vi "SPARK Set Parameter Byte Array.vi"(8 "error in (no error)":errorcluster, 9 "Bytes LSB First":u8[](array[numeric]), 10 "Parameter ID":T6, 11 "MotorControlDeviceRef":T1={"DeviceStatus"={"status"=FALSE, "code"=0, "source"=""}, "Type"=enum."CAN", "PWM"={"PWM Channel"=enum."Invalid", "DeadBand"={"Name"="", "maxPositivePwm"=0, "minPositivePwm"=0, "centerPwm"=0, "maxNegativePwm"=0, "minNegativePwm"=0, "angularRange"=0}}, "CAN"={"Device Number"=8, "SetOutput VI Ref"=variant, "GetOutput VI Ref"=variant, "Enable VI Ref"=variant, "Disable VI Ref"=variant, "Data"=variant(cluster{"Ext ID":u32, "Motor Type":enum16{"Brushed", "Brushless"}} {"Ext ID"=33882120, "Motor Type"=enum."Brushed"})}, "Invert"=FALSE, "DIO PWM"={"PWM \"Enable\" Channel"=enum."Invalid", "DIOChannel"=enum."Invalid", "PWM Rate"=0.0}}) -> (0 "error out":errorcluster, 3 "MotorControlDeviceRef":T1={"DeviceStatus"={"status"=FALSE, "code"=0, "source"=""}, "Type"=enum."CAN", "PWM"={"PWM Channel"=enum."Invalid", "DeadBand"={"Name"="", "maxPositivePwm"=0, "minPositivePwm"=0, "centerPwm"=0, "maxNegativePwm"=0, "minNegativePwm"=0, "angularRange"=0}}, "CAN"={"Device Number"=8, "SetOutput VI Ref"=variant, "GetOutput VI Ref"=variant, "Enable VI Ref"=variant, "Disable VI Ref"=variant, "Data"=variant(cluster{"Ext ID":u32, "Motor Type":enum16{"Brushed", "Brushless"}} {"Ext ID"=33882120, "Motor Type"=enum."Brushed"})}, "Invert"=FALSE, "DIO PWM"={"PWM \"Enable\" Channel"=enum."Invalid", "DIOChannel"=enum."Invalid", "PWM Rate"=0.0}})   [LabVIEW 2023]
uses:
  Typedef/SPARK Parameter ID.ctl
  <vilib>/Rock Robotics/WPI/MotorControl/WPI_MotorControlDeviceRef.ctl
  <vilib>/Rock Robotics/WPI/MotorControl/WPI_MotorControlType.ctl
  <vilib>/Rock Robotics/SystemInterfaces/DIO/FPGA_DIOPWMChannel.ctl
  <vilib>/Rock Robotics/WPI/PWM/WPI_PWMDeadband.ctl
  <vilib>/Rock Robotics/SystemInterfaces/DIO/FPGA_DIOChannel.ctl
  Typedef/Spark MAX Variant Data.ctl
  Typedef/SPARK Model.ctl
  Typedef/SPARK CAN Arb ID.ctl
  Typedef/Spark MAX Parameter Status.ctl
  <vilib>/Utility/error.llb/Error Cluster From Error Code.vi
  <vilib>/ErrorRing/Error Ring.xnode
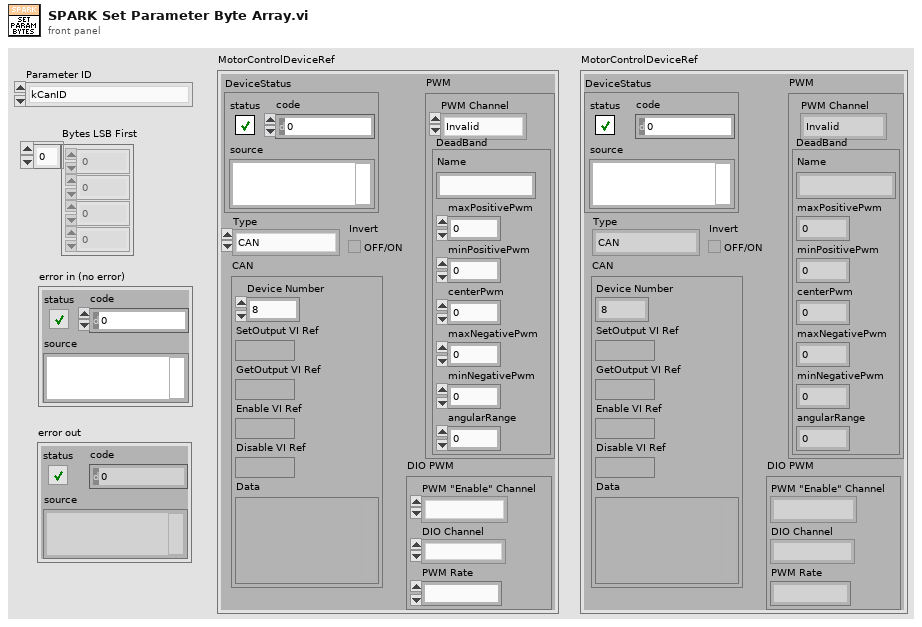
[diagram p1: front panel]
types:
  T1 = typedef "WPI_MotorControlDeviceRef.ctl" = cluster{"DeviceStatus":errorcluster, "Type":T2, "PWM":cluster{"PWM Channel":T3, "DeadBand":T4}, "CAN":cluster{"Device Number":u8, "SetOutput VI Ref":variant, "GetOutput VI Ref":variant, "Enable VI Ref":variant, "Disable VI Ref":variant, "Data":variant}, "Invert":bool, "DIO PWM":cluster{"PWM \"Enable\" Channel":T3, "DIOChannel":T5, "PWM Rate":dbl}}
  T2 = typedef "WPI_MotorControlType.ctl" = enum16{"PWM", "CAN", "DIO PWM"}
  T3 = typedef "FPGA_DIOPWMChannel.ctl" = enum8{"PWM 0", "PWM 1", "PWM 2", "PWM 3", "PWM 4", "PWM 5", "PWM 6", "PWM 7", "PWM 8", "PWM 9", "PWM MXP 0", "PWM MXP 1", "PWM MXP 2", "PWM MXP 3", "PWM MXP 4", "PWM MXP 5", "PWM MXP 6", "PWM MXP 7", "PWM MXP 8", "PWM MXP 9", "Invalid"}
  T4 = typedef "WPI_PWMDeadband.ctl" = cluster{"Name":string, "maxPositivePwm":i32, "minPositivePwm":i32, "centerPwm":i32, "maxNegativePwm":i32, "minNegativePwm":i32, "angularRange":u16}
  T5 = typedef "FPGA_DIOChannel.ctl" = enum8{"DIO 0", "DIO 1", "DIO 2", "DIO 3", "DIO 4", "DIO 5", "DIO 6", "DIO 7", "DIO 8", "DIO 9", "DIO MXP 0", "DIO MXP 1", "DIO MXP 2", "DIO MXP 3", "DIO MXP 4", "DIO MXP 5", "DIO MXP 6", "DIO MXP 7", "DIO MXP 8", "DIO MXP 9", "DIO MXP 10", "DIO MXP 11", "DIO MXP 12", "DIO MXP 13", "DIO MXP 14", "DIO MXP 15", "SPI Port CS1", "SPI Port CS2", "SPI Port CS3", "SPI Port MISO", "SPI Port MOSI", "Invalid"}
  T6 = typedef "SPARK Parameter ID.ctl" = enum16{"kCanID", "kInputMode", "kMotorType", "kCommAdvance", "kSensorType", "kCtrlType", "kIdleMode", "kInputDeadband", "kLegacyFeedbackSensorPID0", "kClosedLoopControlSensor", "kPolePairs", "kCurrentChop", "kCurrentChopCycles", "kP_0", "kI_0", "kD_0", "kF_0", "kIZone_0", "kDFilter_0", "kOutputMin_0", "kOutputMax_0", "kP_1", "kI_1", "kD_1", "kF_1", "kIZone_1", "kDFilter_1", "kOutputMin_1", "kOutputMax_1", "kP_2", "kI_2", "kD_2", "kF_2", "kIZone_2", "kDFilter_2", "kOutputMin_2", "kOutputMax_2", "kP_3", "kI_3", "kD_3", "kF_3", "kIZone_3", "kDFilter_3", "kOutputMin_3", "kOutputMax_3", "kInverted", "kOutputRatio", "kSerialNumberLow", "kSerialNumberMid", "kSerialNumberHigh", "kLimitSwitchFwdPolarity", "kLimitSwitchRevPolarity", "kHardLimitFwdEn", "kHardLimitRevEn", "kSoftLimitFwdEn", "kSoftLimitRevEn", "kRampRate", "kFollowerID", "kFollowerConfig", "kSmartCurrentStallLimit", "kSmartCurrentFreeLimit", "kSmartCurrentConfig", "kSmartCurrentReserved", "kMotorKv", "kMotorR", "kMotorL", "kMotorRsvd1", "kMotorRsvd2", "kMotorRsvd3", "kEncoderCountsPerRev", "kEncoderAverageDepth", "kEncoderSampleDelta", "kEncoderInverted", "kEncoderRsvd1", "kClosedLoopVoltageMode", "kCompensatedNominalVoltage", "kSmartMotionMaxVelocity_0", "kSmartMotionMaxAccel_0", "kSmartMotionMinVelOutput_0", "kSmartMotionAllowedClosedLoopError_0", "kSmartMotionAccelStrategy_0", "kSmartMotionMaxVelocity_1", "kSmartMotionMaxAccel_1", "kSmartMotionMinVelOutput_1", "kSmartMotionAllowedClosedLoopError_1", "kSmartMotionAccelStrategy_1", "kSmartMotionMaxVelocity_2", "kSmartMotionMaxAccel_2", "kSmartMotionMinVelOutput_2", "kSmartMotionAllowedClosedLoopError_2", "kSmartMotionAccelStrategy_2", "kSmartMotionMaxVelocity_3", "kSmartMotionMaxAccel_3", "kSmartMotionMinVelOutput_3", "kSmartMotionAllowedClosedLoopError_3", "kSmartMotionAccelStrategy_3", "kIMaxAccum_0", "kSlot3Placeholder1_0", "kSlot3Placeholder2_0", "kSlot3Placeholder3_0", "kIMaxAccum_1", "kSlot3Placeholder1_1", "kSlot3Placeholder2_1", "kSlot3Placeholder3_1", "kIMaxAccum_2", "kSlot3Placeholder1_2", "kSlot3Placeholder2_2", "kSlot3Placeholder3_2", "kIMaxAccum_3", "kSlot3Placeholder1_3", "kSlot3Placeholder2_3", "kSlot3Placeholder3_3", "kPositionConversionFactor", "kVelocityConversionFactor", "kClosedLoopRampRate", "kSoftLimitFwd", "kSoftLimitRev", "kSoftLimitRsvd0", "kSoftLimitRsvd1", "kAnalogPositionConversion", "kAnalogVelocityConversion", "kAnalogAverageDepth", "kAnalogSensorMode", "kAnalogInverted", "kAnalogSampleDelta", "kAnalogRsvd0", "kAnalogRsvd1", "kDataPortConfig", "kAltEncoderCountsPerRev", "kAltEncoderAverageDepth", "kAltEncoderSampleDelta", "kAltEncoderInverted", "kAltEncoderPositionConversion", "kAltEncoderVelocityConversion", "kAltEncoderRsvd0", "kAltEncoderRsvd1", "kHallSensorSampleRate", "kHallSensorAverageDepth", "kNumParameters", "kDutyCyclePositionFactor", "kDutyCycleVelocityFactor", "kDutyCycleInverted", "kDutyCycleSensorMode", "kDutyCycleAverageDepth", "kDutyCycleSampleDelta", "kDutyCycleOffsetv1p6p2", "kDutyCycleRsvd0", "kDutyCycleRsvd1", "kDutyCycleRsvd2", "kPositionPIDWrapEnable", "kPositionPIDMinInput", "kPositionPIDMaxInput", "kDutyCycleZeroCentered", "kDutyCyclePrescalar", "kDutyCycleOffset", "kProductId", "kDeviceMajorVersion", "kDeviceMinorVersion", "kStatus0Period", "kStatus1Period", "kStatus2Period", "kStatus3Period", "kStatus4Period", "kStatus5Period", "kStatus6Period", "kStatus7Period", "kMAXMotionMaxVelocity_0", "kMAXMotionMaxAccel_0", "kMAXMotionMaxJerk_0", "kMAXMotionAllowedClosedLoopError_0", "kMAXMotionPositionMode_0", "kMAXMotionMaxVelocity_1", "kMAXMotionMaxAccel_1", "kMAXMotionMaxJerk_1", "kMAXMotionAllowedClosedLoopError_1", "kMAXMotionPositionMode_1", "kMAXMotionMaxVelocity_2", "kMAXMotionMaxAccel_2", "kMAXMotionMaxJerk_2", "kMAXMotionAllowedClosedLoopError_2", "kMAXMotionPositionMode_2", "kMAXMotionMaxVelocity_3", "kMAXMotionMaxAccel_3", "kMAXMotionMaxJerk_3", "kMAXMotionAllowedClosedLoopError_3", "kMAXMotionPositionMode_3", "kForceEnableStatus0", "kForceEnableStatus1", "kForceEnableStatus2", "kForceEnableStatus3", "kForceEnableStatus4", "kForceEnableStatus5", "kForceEnableStatus6", "kForceEnableStatus7", "kFollowerModeLeaderId", "kFollowerModeIsInverted", "kDutyCycleEncoderStartPulseUs", "kDutyCycleEncoderEndPulseUs"}
  T7 = typedef "SPARK CAN Arb ID.ctl" = u32
  T8 = typedef "Spark MAX Variant Data.ctl" = cluster{"Ext ID":u32, "CAN Timeout":u32, "Inverted No WPILib":bool, "Has Configured Limit Sw":bool, "Has Configured Alt Encoder":bool, "SPARK Model":T9, "CAN Max Retries":u32, "CAN Timeout (ms)":u32, "Status 0 Period (ms)":u32, "Status 1 Period (ms)":u32, "Status 2 Period (ms)":u32, "Status 3 Period (ms)":u32, "Status 4 Period (ms)":u32, "Status 5 Period (ms)":u32, "Status 6 Period (ms)":u32, "Status 7 Period (ms)":u32, "Status Frame Timeout (ms)":u32}
  T9 = typedef "SPARK Model.ctl" = enum16{"SPARK MAX", "SPARK Flex", "Unknown"}
  T10 = typedef "Spark MAX Parameter Status.ctl" = enum16{"Ok", "Invalid Parameter ID", "Mismatch Type", "Access Mode", "Invalid Parameter Value", "Not Implemented/Depcrecated"}
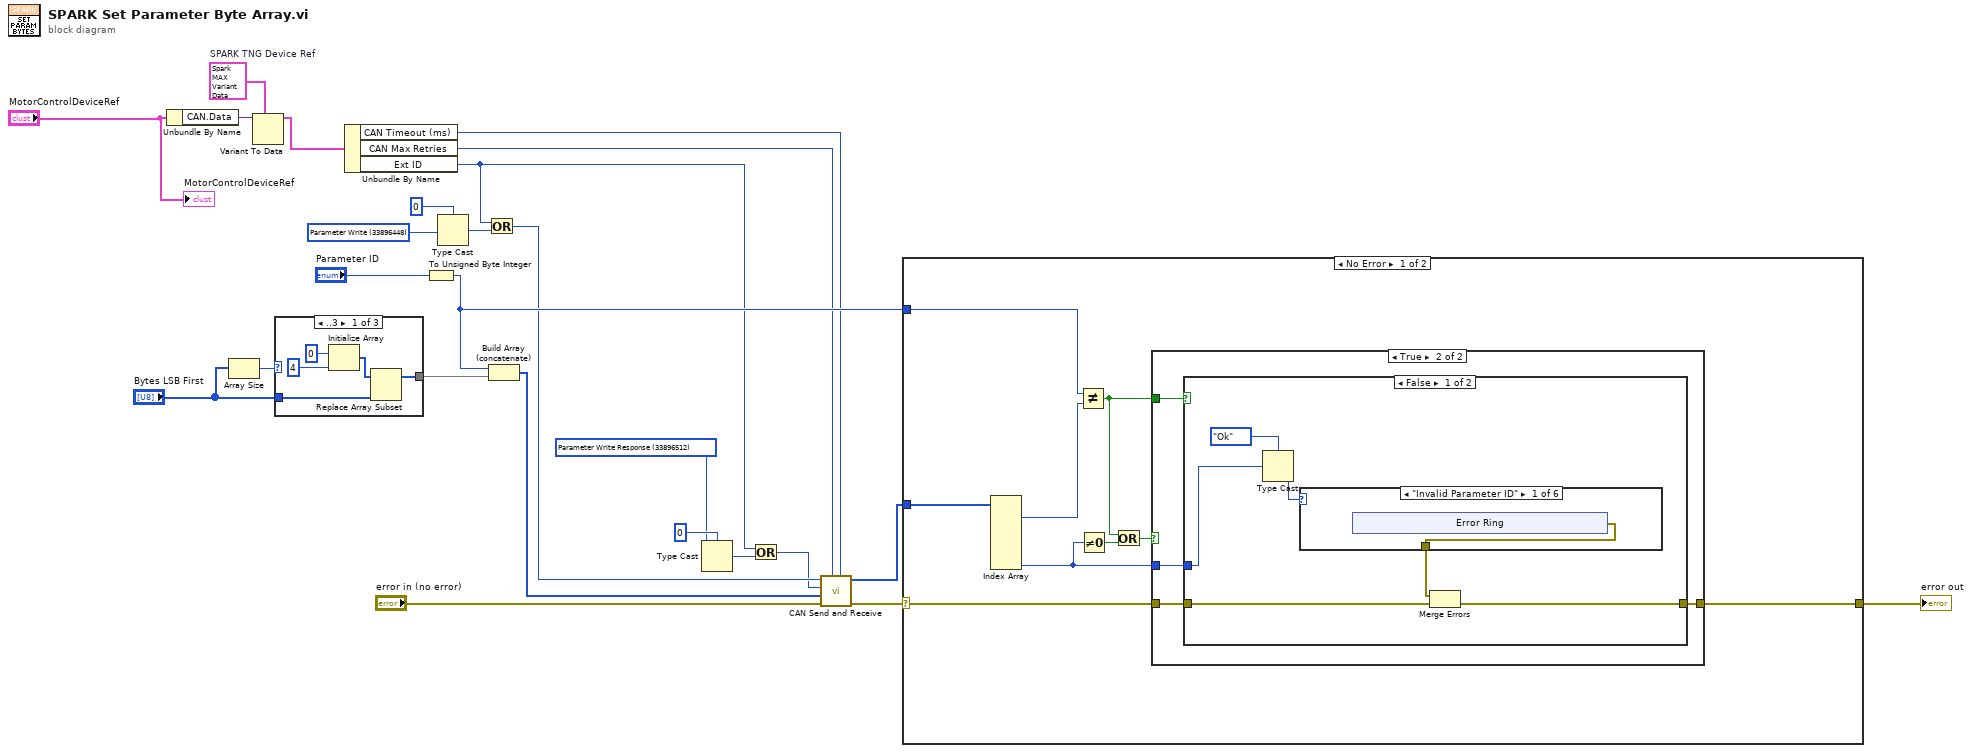
[diagram p0: block diagram]
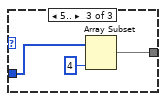
[diagram p3: hidden frame]
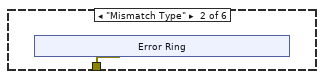
[diagram p5: hidden frame]
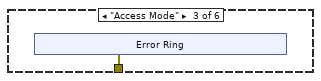
[diagram p6: hidden frame]
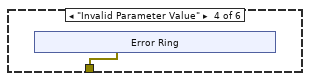
[diagram p7: hidden frame]
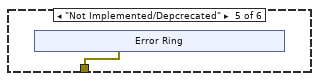
[diagram p8: hidden frame]
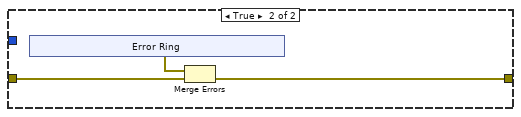
[diagram p10: hidden frame]
diagram:
  w6 = T7 33896512 items=["Broadcast Disable"=0, "Broadcast System Halt"=64, "Broadcast System Reset"=128, "Broadcast Device Assign"=192, "Broadcast Heartbeat"=320, "Broadcast Firmware Version"=512, "Broadcast Enumerate"=576, "Broadcast System Resume"=640, "Velocity Setpoint"=33882112, "Duty Cycle Setpoint"=33882240, "Smart Velocity Setpoint"=33882304, "Position Setpoint"=33882368, "Voltage Setpoint"=33882432, "Current Setpoint"=33882496, "Smart Motion Setpoint"=33882560, "MAXMotion Position Setpoint"=33882624, "MAXMotion Velocity Setpoint"=33882688, "Periodic Status 0"=33929216, "Periodic Status 1"=33929280, "Periodic Status 2"=33929344, "Periodic Status 3"=33929408, "Periodic Status 4"=33929472, "Periodic Status 5"=33929536, "Periodic Status 6"=33929600, "Periodic Status 7"=33929664, "DRV Status"=33888896, "Clear Faults"=33889152, "Parameter Write"=33896448, "Parameter Write Response"=33896512, "Get Config Parameter"=33889344, "Config Burn Flash"=33889408, "Set Follower Mode"=33889472, "Config Factory Defaults"=33889536, "Config Factory Reset"=33889600, "Nack"=33890304, "Ack"=33890368, "Broadcast (not a command)"=33891328, "Heartbeat"=33891456, "Sync"=33891520, "IDQuery"=33891584, "IDAssign"=33891648, "Firmware Version"=33891840, "REV Enumerate"=33891904, "Legacy/USB Heartbeat"=33891968, "roboRIO Lock"=33892032, "SWDL Data"=33892096, "SWDL Checksum"=33892160, "SWDL Retransmit"=33892224, "Telemetry Update Mechanical Position Enoder Port"=33892352, "Telemetry Update I Accum"=33892480, "Telemtry Update Mechanical Position Alt Encoder"=33892608, "Telemetry Update Mechanical Position Analog"=33892544, "Non-roboRIO Broadcast (not a command)"=33893376, "non-RIO Lock"=33893440, "non-RIO Heartbeat"=33893504] ("SPARK Arb ID")
  w14 = T7 33896448 items=["Broadcast Disable"=0, "Broadcast System Halt"=64, "Broadcast System Reset"=128, "Broadcast Device Assign"=192, "Broadcast Heartbeat"=320, "Broadcast Firmware Version"=512, "Broadcast Enumerate"=576, "Broadcast System Resume"=640, "Velocity Setpoint"=33882112, "Duty Cycle Setpoint"=33882240, "Smart Velocity Setpoint"=33882304, "Position Setpoint"=33882368, "Voltage Setpoint"=33882432, "Current Setpoint"=33882496, "Smart Motion Setpoint"=33882560, "MAXMotion Position Setpoint"=33882624, "MAXMotion Velocity Setpoint"=33882688, "Periodic Status 0"=33929216, "Periodic Status 1"=33929280, "Periodic Status 2"=33929344, "Periodic Status 3"=33929408, "Periodic Status 4"=33929472, "Periodic Status 5"=33929536, "Periodic Status 6"=33929600, "Periodic Status 7"=33929664, "DRV Status"=33888896, "Clear Faults"=33889152, "Parameter Write"=33896448, "Parameter Write Response"=33896512, "Get Config Parameter"=33889344, "Config Burn Flash"=33889408, "Set Follower Mode"=33889472, "Config Factory Defaults"=33889536, "Config Factory Reset"=33889600, "Nack"=33890304, "Ack"=33890368, "Broadcast (not a command)"=33891328, "Heartbeat"=33891456, "Sync"=33891520, "IDQuery"=33891584, "IDAssign"=33891648, "Firmware Version"=33891840, "REV Enumerate"=33891904, "Legacy/USB Heartbeat"=33891968, "roboRIO Lock"=33892032, "SWDL Data"=33892096, "SWDL Checksum"=33892160, "SWDL Retransmit"=33892224, "Telemetry Update Mechanical Position Enoder Port"=33892352, "Telemetry Update I Accum"=33892480, "Telemtry Update Mechanical Position Alt Encoder"=33892608, "Telemetry Update Mechanical Position Analog"=33892544, "Non-roboRIO Broadcast (not a command)"=33893376, "non-RIO Lock"=33893440, "non-RIO Heartbeat"=33893504] ("SPARK Arb ID")
  w24 = T8 {"Ext ID"=0, "CAN Timeout"=0, "Inverted No WPILib"=FALSE, "Has Configured Limit Sw"=FALSE, "Has Configured Alt Encoder"=FALSE, "SPARK Model"=enum."Unknown", "CAN Max Retries"=5, "CAN Timeout (ms)"=20, "Status 0 Period (ms)"=10, "Status 1 Period (ms)"=250, "Status 2 Period (ms)"=20, "Status 3 Period (ms)"=20, "Status 4 Period (ms)"=20, "Status 5 Period (ms)"=20, "Status 6 Period (ms)"=20, "Status 7 Period (ms)"=20, "Status Frame Timeout (ms)"=500}  # SPARK TNG Device Ref
  n1 = Unbundle By Name("MotorControlDeviceRef") -> ("CAN.Data"=w25:variant)
  n2 = Array Size(array="Bytes LSB First") -> (size(s)=w18:i32)
  n3 = Variant To Data(type=w24, Variant=w25) -> (data=w15:T8)  [unwired: 1 in, 1 out]
  n4 = case shown="..3" w18 {
    tunnel: "Bytes LSB First" -> [w28 w31 w34]
    tunnel: [w26 w31 w32] -> w13
    frame ..3 {
      n5 = Initialize Array(u8 0 ("element"), 4 ("dimension size")) -> (w29:u8[])
      n6 = Replace Array Subset(array=w29, new element=w28) -> (w26:u8[])  [unwired: 1 in]
    }
    frame 4 {
    }
    frame 5.. {
      n7 = Array Subset(array=w34, length=4) -> (w32:u8[])  [unwired: 1 in]
    }
  }
  n8 = Unbundle By Name(w15) -> ("CAN Timeout (ms)"=w2:u32, "CAN Max Retries"=w3:u32, "Ext ID"=w5:u32)
  n9 = To Unsigned Byte Integer(number="Parameter ID") -> (unsigned 8bit integer=w17:u8)
  n10 = Type Cast(type=u32 0 ("element"), x=w14) -> (*(type *) &x=w23:u32)
  n11 = Or(x=w5, y=w23) -> (x .or. y?=w9:u32)
  n12 = Build Array (concatenate)(w17, w13) -> (w10:u8[])
  n13 = Type Cast(type=u32 0 ("element"), x=w6) -> (*(type *) &x=w8:u32)
  n14 = Or(x=w5, y=w8) -> (x .or. y?=w4:u32)
  n15 = call "CAN Send and Receive.vi"("CAN Timeout (ms)"=w2, "CAN Max Retries"=w3, "error in (no error)"="error in (no error)", "Send Data"=w10, "Receive Message ID"=w4, "Send Message ID"=w9) -> ("error out"=w11:errorcluster, "Receive Data"=w1:u8[])  [unwired: 4 in]
  n16 = case shown="No Error" w11 {
    selector: w11 -> [w36 w87]
    tunnel: w17 -> [w43 _]
    tunnel: [w42 w87] -> w16
    tunnel: w1 -> [w41 _]
    frame No Error {
      n17 = Index Array(array=w41) -> (element #1=w40:u8, element #7=w35:u8)  [unwired: 7 in, 5 out]
      n18 = Not Equal?(x=w43, y=w40) -> (x != y?=w37:bool)
      n19 = Not Equal To 0?(x=w35) -> (x != 0?=w39:bool)
      n20 = Or(x=w37, y=w39) -> (x .or. y?=w38:bool)
      n21 = case shown="True" w38 {
        tunnel: [w44 w47] -> w42
        tunnel: w36 -> [w44 w48]
        tunnel: w37 -> [_ w46]
        tunnel: w35 -> [_ w45]
        frame False {
        }
        frame True {
          n22 = case shown="False" w46 {
            tunnel: w48 -> [w54 w82]
            tunnel: [w53 w81] -> w47
            tunnel: w45 -> [w51 _]
            frame False {
              n23 = Type Cast(type=Spark_MAX_Parameter_Status."Ok" ("Parameter Status"), x=w51) -> (*(type *) &x=w50:T10)
              n24 = case shown="\"Invalid Parameter ID\"" w50 {
                tunnel: [w55 w60 w65 w70 w75 _] -> w49
                frame "Invalid Parameter ID" {
                  n25 = xnode "Error Ring"() -> ("error out"=w55:errorcluster)
                }
                frame "Mismatch Type" {
                  n26 = xnode "Error Ring"() -> ("error out"=w60:errorcluster)
                }
                frame "Access Mode" {
                  n27 = xnode "Error Ring"() -> ("error out"=w65:errorcluster)
                }
                frame "Invalid Parameter Value" {
                  n28 = xnode "Error Ring"() -> ("error out"=w70:errorcluster)
                }
                frame "Not Implemented/Depcrecated" {
                  n29 = xnode "Error Ring"() -> ("error out"=w75:errorcluster)
                }
                frame "Ok", Default {
                }
              }
              n30 = Merge Errors(w49, w54) -> (w53:errorcluster)
            }
            frame True {
              n31 = xnode "Error Ring"() -> ("error out"=w80:errorcluster)
              n32 = Merge Errors(w80, w82) -> (w81:errorcluster)
            }
          }
        }
      }
    }
    frame Error {
    }
  }
  "error out" <- w16
  "MotorControlDeviceRef" <- "MotorControlDeviceRef"
